vi "GT Pvt Table Percent.vi"(0 "cardNum":i16, 1 "pPos":dbl[](array[numeric]), 2 "velBegin":dbl, 5 "tableId":i16, 7 "count":i32, 9 "pTime":dbl[](array[numeric]), 11 "error in (no error)":errorcluster caption="错误输入（无错误）", 12 "pPercent":dbl[](array[numeric])) -> (3 "pPos out":dbl[](array[numeric]), 4 "function return":i16, 10 "pTime out":dbl[](array[numeric]), 14 "pPercent out":dbl[](array[numeric]), 15 "error out":errorcluster caption="错误输出")   [LabVIEW 2020, in "gts.lvlib"]
doc: "GT_API GT_PvtTablePercent(short cardNum,short tableId,long count,double *pTime,double *pPos,double *pPercent,double velBegin=0);"
uses:
  gts.lvlib
  dll/32bit/multi_card/gts.dll
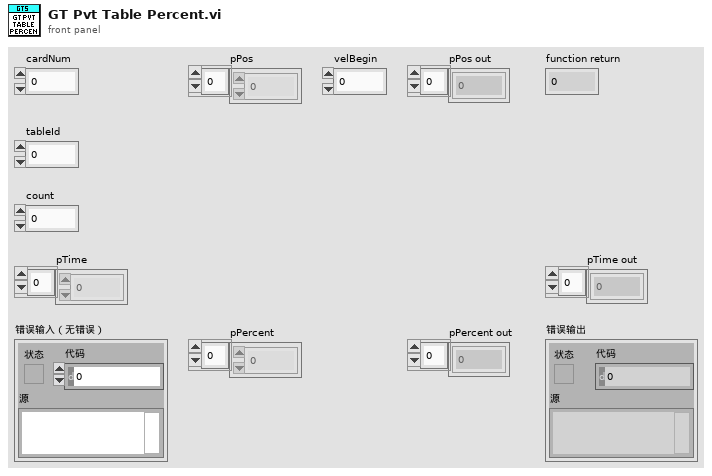
[diagram p1: front panel]
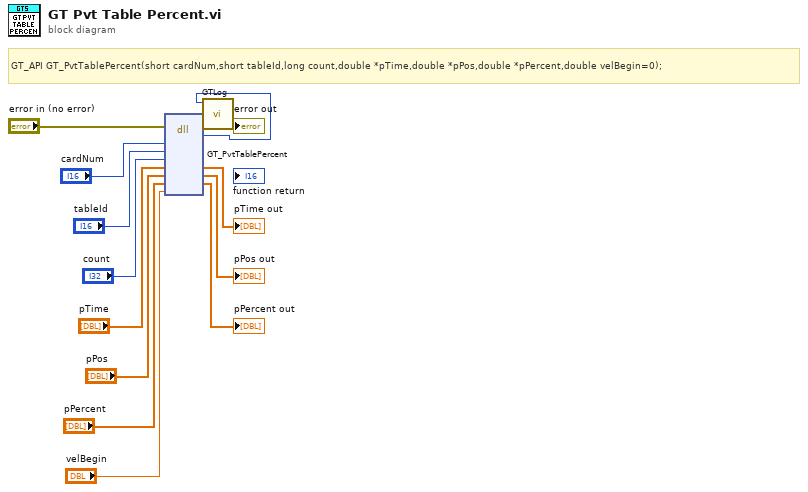
[diagram p0: block diagram]
diagram:
  # "GT_API GT_PvtTablePercent(short cardNum,short tableId,long count,double *pTime,double *pPos,double *pPercent,double velBegin=0);"
  n1 = dll-call lib="C:/1228/dll/32bit/multi_card/gts.dll" fn="GT_PvtTablePercent"(error in="error in (no error)", "cardNum"="cardNum", "tableId"="tableId", "count"="count", "pTime"="pTime", "pPos"="pPos", "pPercent"="pPercent", "velBegin"="velBegin") -> (error out=w3:errorcluster, "返回类型"=w1:i16, "pTime"=→"pTime out":dbl[], "pPos"=→"pPos out":dbl[], "pPercent"=→"pPercent out":dbl[])  [unwired: 6 in, 1 out]
  n2 = call "GTLog.vi"("error in (no error)"=w3, "Numeric"=w1) -> ("error out"=→"error out":errorcluster)  [unwired: 9 in]
